vi "browseVariant.vi"(4 "Variant":variant caption="Value", 5 "Name":string, 6 "error in (no error)":errorcluster, 7 "ParentTag":string, 9 "VariantProbe.lvclass in":refnum<class "Failures_VariantTree__VP.lvclass">) -> (0 "error out":errorcluster, 3 "VariantProbe.lvclass out":refnum<class "Failures_VariantTree__VP.lvclass">)   [LabVIEW 2013, in "Failures_VariantTree__VP.lvclass"]
uses:
  Failures_VariantTree__VP.lvclass
  Failures_VariantTree__VP.lvclass/Failures_VariantTree__VP.ctl
  <vilib>/Utility/VariantDataType/VariantType.lvlib
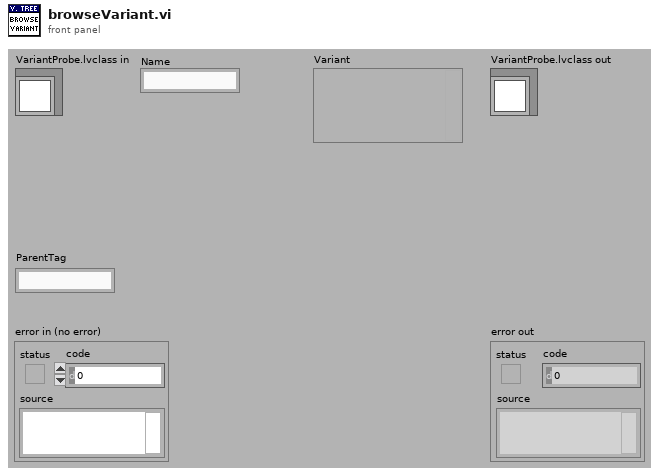
[diagram p1: front panel]
types:
  T1 = typedef "Type Descriptor Enumeration__ogtk.ctl" = enum8{"<Null>", "I8", "I16", "I32", "I64", "U8", "U16", "U32", "U64", "SGL", "DBL", "EXT", "CSG", "CDB", "CXT", "0x0F", "0x10", "0x11", "0x12", "0x13", "0x14", "Enum U8", "Enum U16", "Enum U32", "Enum U64", "SGL PQ", "DBL PQ", "EXT PQ", "CSG PQ", "CDB PQ", "CXT PQ", "0x1F", "0x20", "Boolean", "0x22", "0x23", "0x24", "0x25", "0x26", "0x27", "0x28", "0x29", "0x2A", "0x2B", "0x2C", "0x2D", "0x2E", "0x2F", "String", "0x31", "Path", "Pict", "0x34", "0x35", "0x36", "DAQ", "0x38", "0x39", "0x3A", "0x3B", "0x3C", "0x3D", "0x3E", "0x3F", "Array", "0x41", "0x42", "0x43", "0x44", "0x45", "0x46", "0x47", "0x48", "0x49", "0x4A", "0x4B", "0x4C", "0x4D", "0x4E", "0x4F", "Cluster", "0x51", "0x52", "Variant", "Waveform", "0x55", "0x56", "0x57", "0x58", "0x59", "0x5A", "0x5B", "0x5C", "0x5D", "0x5E", "0x5F", "0x60", "0x61", "0x62", "0x63", "0x64", "0x65", "0x66", "0x67", "0x68", "0x69", "0x6A", "0x6B", "0x6C", "0x6D", "0x6E", "0x6F", "Refnum"}
  T2 = typedef "Type Descriptor Header__ogtk.ctl" = cluster{"length":u16, "private":u8, "type":T1, "# elements":u16}
  T3 = typedef "Physical Units__ogtk.ctl" = cluster{"Base Units":enum16{"radian", "steradian", "second", "meter", "kilogram", "ampere", "kelvin", "mole", "candela"}, "Exponent":i16}
  T4 = enum16{"radian", "steradian", "second", "meter", "kilogram", "ampere", "kelvin", "mole", "candela"}
  T5 = typedef "VariantType.lvlib/RefnumType.ctl" = enum16{"NotARefnum", "UnknownRefnum", "Generic", "Datalog", "ByteStream", "Device", "Occurence", "TCPNetConnection", "Auto", "Menu", "Imaq", "Hardware", "DataSocket", "Visa", "IVI", "UDPNetConnection", "Notifier", "Queue", "Irda", "EventReg", "DotNet", "UserEvent", "Callback", "UNUSED_EMPTY_POSITION", "BlueToothNetConnection", "LVObjApp", "LVObjVI", "LVObjUnknown", "GenericClass", "UserDefinedRefnumTag", "DataValue", "RT FIFO", "TDMS File"}
  T6 = enum32{"invalid VI type", "Standard VI", "Control VI", "Global VI", "Polymorphic VI", "Configuration VI", "SubSystem", "Facade VI", "Method VI", "Statechart Diagram VI"}
  T7 = typedef "VariantType.lvlib/Type.ctl" = enum8{"Invalid Type", "Void", "I8", "I16", "I32", "I64", "U8", "U16", "U32", "U64", "Single Float", "Double Float", "Extended Float", "Single Complex", "Double Complex", "Extended Complex", "Enum U8", "Enum U16", "Enum U32", "Enum U64", "Single Float With Unit", "Double Float With Unit", "Extended Float With Unit", "Single Complex with Unit", "Double Complex with Unit", "Extended Complex with Unit", "Boolean", "String", "Path", "Picture", "Tag", "Array", "Cluster", "Variant", "LV Variant", "Waveform", "Timestamp", "Digital Waveform", "Digital Data", "ExpressData", "Refnum", "External Data", "VI", "Poly VI", "LabVIEW Class Instance", "Fixed Point"}
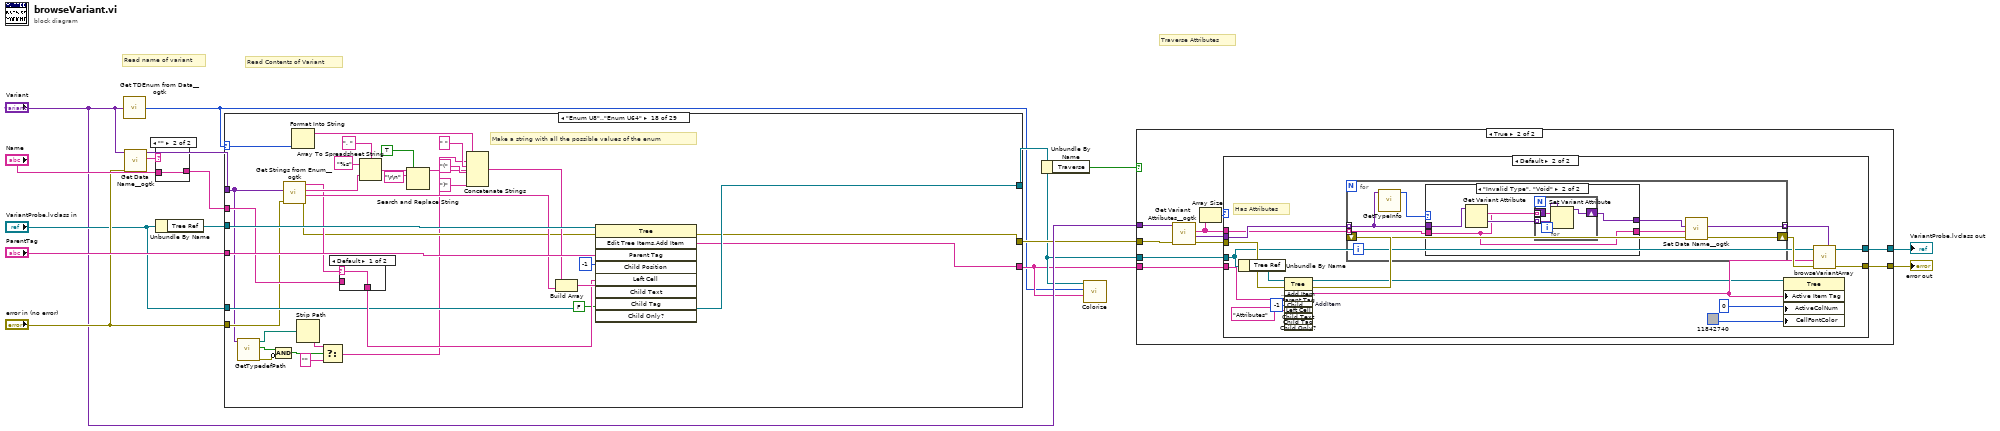
[diagram p0: block diagram]
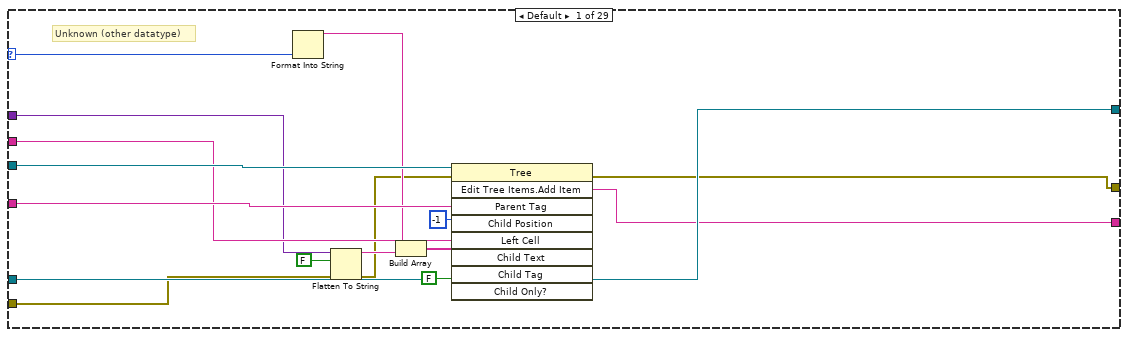
[diagram p6: hidden frame]
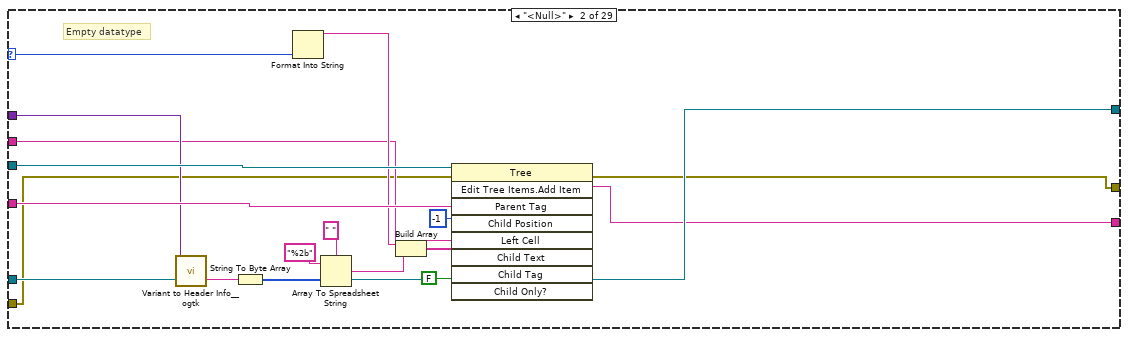
[diagram p7: hidden frame]
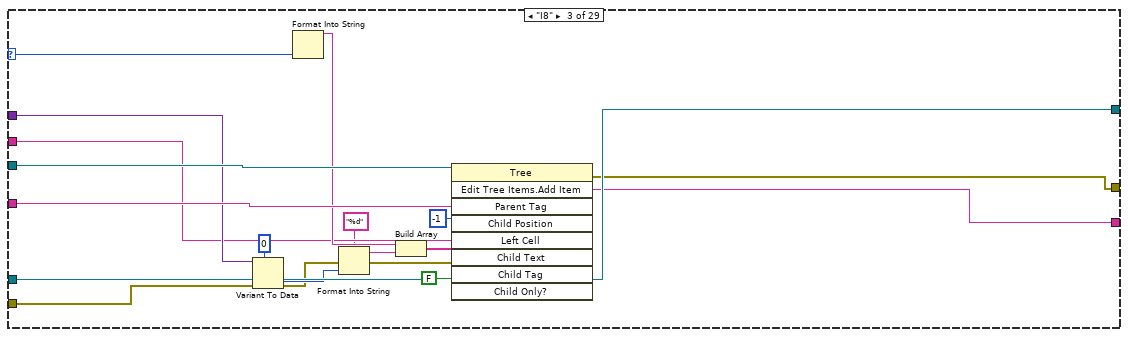
[diagram p8: hidden frame]
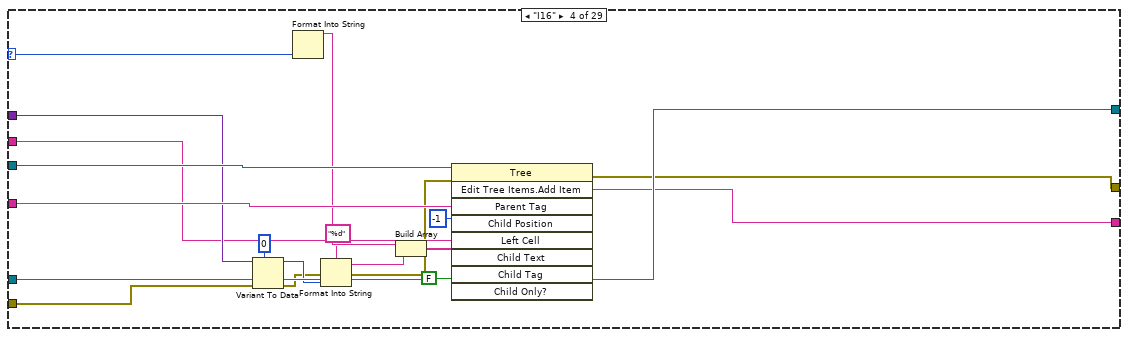
[diagram p9: hidden frame]
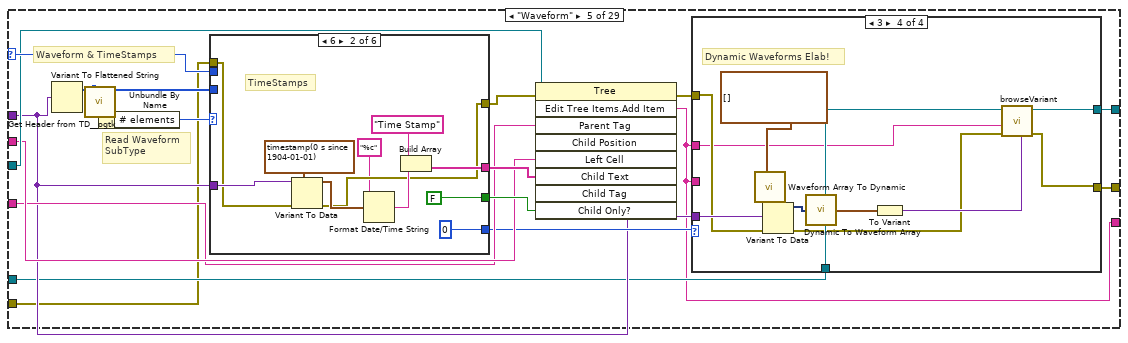
[diagram p10: hidden frame]
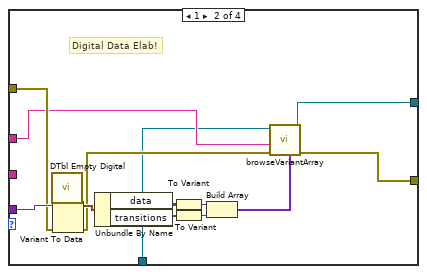
[diagram p12: hidden frame]
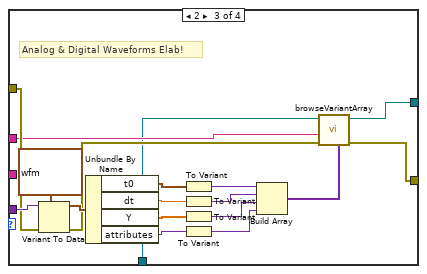
[diagram p13: hidden frame]
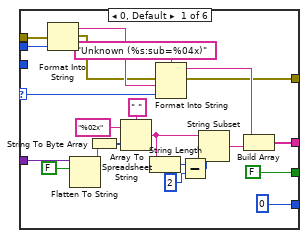
[diagram p14: hidden frame]
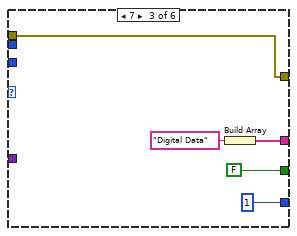
[diagram p15: hidden frame]
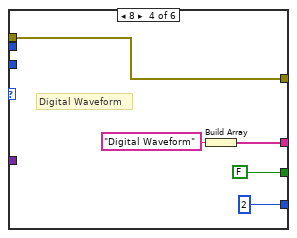
[diagram p16: hidden frame]
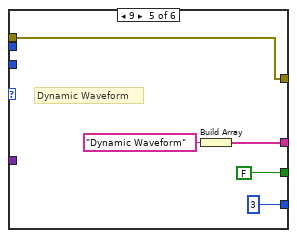
[diagram p17: hidden frame]
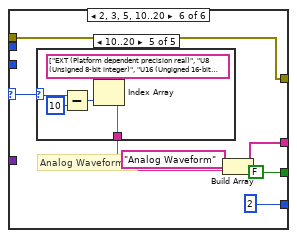
[diagram p18: hidden frame]
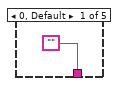
[diagram p19: hidden frame]
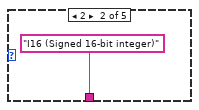
[diagram p20: hidden frame]
diagram:
  # "Traverse Attributes"
  # "Read Contents of Variant"
  # "Read name of variant"
  n1 = call <userlib>:"Get TDEnum from Data__ogtk.vi"("Data"="Variant") -> ("Type Descriptor Enumeration"=w1:T1)  [unwired: 4 in]
  n2 = call <userlib>:"Get Data Name__ogtk.vi"("error in (no error)"="error in (no error)", "Data"="Variant") -> ("Data Name"=w16:string, "Data dup"=w14:variant)  [unwired: 7 in, 1 out]
  n3 = case shown="\"\"" w16 {
    selector: w16 -> [w17 _]
    tunnel: [w17 w18] -> w13
    tunnel: "Name" -> [_ w18]
    frame Default {
    }
    frame "" {
    }
  }
  n4 = Unbundle By Name("VariantProbe.lvclass in") -> ("Tree Ref"=w4:refnum<vi>)
  n5 = case shown="\"Enum U8\"..\"Enum U64\"" w1 {
    selector: w1 -> [w34 w52 w71 w90 w105 w237 w256 w275 w294 w313 w332 w350 w368 w386 w404 w422 w440 w471 w504 w538 w572 w598 w614 w631 w647 _ _ _ w718]
    tunnel: w14 -> [w25 w41 w64 w83 w97 w230 w249 w268 w287 w306 w325 w339 w358 w376 w394 w412 w430 w448 w492 w526 w560 w587 w605 w622 w638 w659 w673 w703 w709]
    tunnel: w4 -> [w31 w49 w68 w87 w104 w234 w253 w272 w291 w310 w329 w347 w365 w383 w401 w419 w437 w475 w501 w535 w569 w595 w611 w628 w644 w669 w684 w708 w716]
    tunnel: "ParentTag" -> [w33 w51 w70 w89 w99 w236 w255 w274 w293 w312 w331 w349 w367 w385 w403 w421 w439 w474 w503 w537 w571 w597 w613 w630 w646 w668 w683 w707 w717]
    tunnel: w13 -> [w26 w40 w63 w82 w100 w229 w248 w267 w286 w305 w324 w340 w357 w375 w393 w411 w429 w457 w495 w529 w563 w586 w606 w621 w639 w660 w680 w702 w714]
    tunnel: "VariantProbe.lvclass in" -> [w23 w38 w61 w80 w96 w227 w246 w265 w284 w303 w322 w337 w355 w373 w391 w409 w427 w453 w485 w519 w553 w584 w603 w619 w636 w650 w678 w697 w713]
    tunnel: [w23 w38 w61 w80 w95 w227 w246 w265 w284 w303 w322 w337 w355 w373 w391 w409 w427 w453 w485 w519 w553 w584 w603 w619 w636 w649 w677 w695 w713] -> w3
    tunnel: "error in (no error)" -> [w22 w37 w59 w78 w94 w226 w244 w264 w283 w301 w321 w335 w354 w372 w390 w408 w425 w452 w484 w518 w552 w582 w601 w616 w635 w656 w675 w700 _]
    tunnel: [w20 w36 w60 w79 w92 w225 w245 w263 w282 w302 w314 w334 w352 w370 w388 w406 w424 w450 w479 w513 w547 w581 w600 w618 w633 w653 w676 w699 w712] -> w8
    tunnel: [w19 w35 w53 w72 w91 w219 w238 w257 w276 w295 w315 w333 w351 w369 w387 w405 w423 w449 w478 w512 w546 w580 w599 w615 w632 w648 w674 w694 w711] -> w2
    frame Default {
      # "Unknown (other datatype)"
      n6 = Format Into String(w34) -> (resulting string=w30:string)  [unwired: 3 in, 1 out]
      n7 = Flatten To String(anything=w25, prepend array or string size? (T)=FALSE, error in (no error)=w22) -> (data string=w28:string, error out=w21:errorcluster)  [unwired: 1 in, 1 out]
      n8 = Build Array(w30, w28) -> (w29:string[])
      n9 = invoke class="Tree" method="Edit Tree Items.Add Item"(reference=w31, error in=w21, "Parent Tag"=w33, "Child Position"=-1, "Left Cell"=w26, "Child Text"=w29, "Child Only?"=FALSE) -> (error out=w20:errorcluster, "Edit Tree Items:Add Item"=w19:string)  [unwired: 2 in, 7 out]
    }
    frame "<Null>" {
      # "Empty datatype"
      n10 = call <userlib>:"Variant to Header Info__ogtk.vi"("Variant"=w41) -> ("data string"=w43:string)  [unwired: 3 in, 2 out]
      n11 = String To Byte Array(string=w43) -> (unsigned byte array=w42:u8[])
      n12 = Format Into String(w52) -> (resulting string=w48:string)  [unwired: 3 in, 1 out]
      n13 = Array To Spreadsheet String(delimiter (Tab)=" ", array=w42, 3:"%2b" ("format string")) -> (spreadsheet string=w44:string)
      n14 = Build Array(w48, w44) -> (w47:string[])
      n15 = invoke class="Tree" method="Edit Tree Items.Add Item"(reference=w49, error in=w37, "Parent Tag"=w51, "Child Position"=-1, "Left Cell"=w40, "Child Text"=w47, "Child Only?"=FALSE) -> (error out=w36:errorcluster, "Edit Tree Items:Add Item"=w35:string)  [unwired: 2 in, 7 out]
    }
    frame "I8" {
      n16 = Variant To Data(error in=w59, type=i8 0, Variant=w64) -> (data=w58:i8, error out=w55:errorcluster)
      n17 = Format Into String(w71) -> (resulting string=w67:string)  [unwired: 3 in, 1 out]
      n18 = Format Into String(format string="%d", error in=w55, w58) -> (resulting string=w57:string, error out=w54:errorcluster)  [unwired: 1 in]
      n19 = Build Array(w67, w57) -> (w66:string[])
      n20 = invoke class="Tree" method="Edit Tree Items.Add Item"(reference=w68, error in=w54, "Parent Tag"=w70, "Child Position"=-1, "Left Cell"=w63, "Child Text"=w66, "Child Only?"=FALSE) -> (error out=w60:errorcluster, "Edit Tree Items:Add Item"=w53:string)  [unwired: 2 in, 7 out]
    }
    frame "I16" {
      n21 = Variant To Data(error in=w78, type=i16 0, Variant=w83) -> (data=w76:i16, error out=w75:errorcluster)
      n22 = Format Into String(w90) -> (resulting string=w86:string)  [unwired: 3 in, 1 out]
      n23 = Format Into String(format string="%d", error in=w75, w76) -> (resulting string=w73:string, error out=w74:errorcluster)  [unwired: 1 in]
      n24 = Build Array(w86, w73) -> (w85:string[])
      n25 = invoke class="Tree" method="Edit Tree Items.Add Item"(reference=w87, error in=w74, "Parent Tag"=w89, "Child Position"=-1, "Left Cell"=w82, "Child Text"=w85, "Child Only?"=FALSE) -> (error out=w79:errorcluster, "Edit Tree Items:Add Item"=w72:string)  [unwired: 2 in, 7 out]
    }
    frame "Waveform" {
      # "Read Waveform\nSubType"
      # "Waveform & TimeStamps"
      n26 = Variant To Flattened String(Variant=w97) -> (1:w108:i16[])  [unwired: 1 out]
      n27 = call <userlib>:"Get Header from TD__ogtk.vi"("Type Descriptor"=w108) -> ("Type Descriptor Header"=w106:T2)
      n28 = Unbundle By Name(w106) -> ("# elements"=w107:u16)
      n29 = case shown="6" w107 {
        selector: w107 -> [w163 _ _ _ _ w208]
        tunnel: [w165 w184 w191 w196 w201 w209] -> w102
        tunnel: w97 -> [w164 w186 _ _ _ _]
        tunnel: w108 -> [_ _ _ _ _ _]
        tunnel: [0 0 1 2 3 2] -> w98
        tunnel: [FALSE ("Child Only?") FALSE ("Child Only?") FALSE ("Child Only?") FALSE ("Child Only?") FALSE ("Child Only?") FALSE ("Child Only?")] -> w101
        tunnel: w105 -> [w159 _ _ _ _ _]
        tunnel: [w157 w178 w188 w193 w198 w203] -> w103
        tunnel: w94 -> [w155 w181 w188 w193 w198 w203]
        frame 0, Default {
          n30 = Format Into String(error in=w155, w159) -> (resulting string=w158:string, error out=w156:errorcluster)  [unwired: 2 in]
          n31 = Flatten To String(anything=w164, prepend array or string size? (T)=FALSE) -> (data string=w166:string)  [unwired: 2 in, 2 out]
          n32 = String To Byte Array(string=w166) -> (unsigned byte array=w160:u8[])
          n33 = Array To Spreadsheet String(delimiter (Tab)=" ", array=w160, 3:"%02x" ("format string")) -> (spreadsheet string=w172:string)
          n34 = String Length(string=w172) -> (length=w173:i32)
          n35 = Format Into String(format string="Unknown (%s:sub=%04x)", error in=w156, w158, w163) -> (resulting string=w169:string, error out=w157:errorcluster)  [unwired: 1 in]
          n36 = Subtract(x=w173, y=2) -> (x-y=w175:i32)
          n37 = String Subset(string=w172, length (rest)=w175) -> (substring=w176:string)  [unwired: 1 in]
          n38 = Build Array(w169, w176) -> (w165:string[])
        }
        frame 6 {
          # "TimeStamps"
          n39 = Variant To Data(error in=w181, type=timestamp(0 s since 1904-01-01), Variant=w186) -> (data=w179:timestamp, error out=w178:errorcluster)
          n40 = Format Date/Time String(time format string (%c)="%c" ("format string"), seconds (now)=w179) -> (date/time string=w180:string)  [unwired: 1 in]
          n41 = Build Array("Time Stamp" ("format string"), w180) -> (w184:string[])
        }
        frame 7 {
          n42 = Build Array("Digital Data" ("format string")) -> (w191:string[])
        }
        frame 8 {
          # "Digital Waveform"
          n43 = Build Array("Digital Waveform" ("format string")) -> (w196:string[])
        }
        frame 9 {
          # "Dynamic Waveform"
          n44 = Build Array("Dynamic Waveform" ("format string")) -> (w201:string[])
        }
        frame 2, 3, 5, 10..20 {
          # "Analog Waveform"
          n45 = case shown="10..20" w208 {
            selector: w208 -> [_ _ _ _ w216]
            tunnel: ["" "I16 (Signed 16-bit integer)" "DBL (Double 64-bit real)" "SGL (Single 32-bit real)" w218] -> w204
            frame 0, Default {
            }
            frame 2 {
            }
            frame 3 {
            }
            frame 5 {
            }
            frame 10..20 {
              n46 = Subtract(x=w216, y=u16 10) -> (x-y=w214:u16)
              n47 = Index Array(array=string[] ["EXT (Platform dependent precision real)", "U8 (Unsigned 8-bit integer)", "U16 (Ungigned 16-bit integer)", "U32 (Unsigned 32-bit integer)", "I8 (Signed 8-bit integer)", "I32 (Signed 32-bit integer)", "CSG (Single 32-bit complex real)", "CDB (Double 64-bit complex real)", "CXT (Extended complex real)", "I64 (Signed 64-bit integer)", "U64 (Unsigned 64-bit integer)"], index=w214) -> (element=w218:string)
            }
          }
          n48 = Build Array("Analog Waveform" ("format string"), w204) -> (w209:string[])
        }
      }
      n49 = invoke class="Tree" method="Edit Tree Items.Add Item"(reference=w104, error in=w103, "Parent Tag"=w99, "Left Cell"=w100, "Child Text"=w102, "Child Only?"=w101) -> (error out=w93:errorcluster, "Edit Tree Items:Add Item"=w91:string)  [unwired: 3 in, 7 out]
      n50 = case shown="3" w98 {
        tunnel: w91 -> [_ w114 w128 w147]
        tunnel: w97 -> [_ w124 w142 w150]
        tunnel: w91 -> [_ _ _ _]
        tunnel: w96 -> [w110 w112 w126 w148]
        tunnel: [w110 w111 w125 w145] -> w95
        tunnel: w93 -> [w109 w117 w131 w149]
        tunnel: [w109 w113 w127 w144] -> w92
        frame 0, Default {
          # "No further elaborations!"
        }
        frame 1 {
          # "Digital Data Elab!"
          n51 = call <vilib>:"DTbl Empty Digital.vi"() -> ("digital data"=w123:digitaldata)  [unwired: 5 in]
          n52 = Variant To Data(error in=w117, type=w123, Variant=w124) -> (data=w122:digitaldata, error out=w116:errorcluster)
          n53 = Unbundle By Name(w122) -> ("data"=w119:u8[][], "transitions"=w118:u32[])
          n54 = To Variant(anything=w119) -> (Variant=w121:variant)
          n55 = To Variant(anything=w118) -> (Variant=w120:variant)
          n56 = Build Array(w121, w120) -> (w115:variant[])
          n57 = call-dynamic "browseVariantArray.vi"("Array of Variants"=w115, "error in"=w116, "ParentTag"=w114, "VariantProbe.lvclass in"=w112) -> ("error out"=w113:errorcluster, "VariantProbe.lvclass out"=w111:refnum<class "Failures_VariantTree__VP.lvclass">)  [unwired: 4 in]
        }
        frame 2 {
          # "Analog & Digital Waveforms Elab!"
          n58 = Variant To Data(error in=w131, type=waveform(dbl) {"t0"=timestamp(0 s since 1904-01-01), "dt"=1.0, "Y"=[]} ("waveform"), Variant=w142) -> (data=w134:waveform(dbl), error out=w129:errorcluster)
          n59 = Unbundle By Name(w134) -> ("t0"=w136:timestamp, "dt"=w138:dbl, "Y"=w137:dbl[], "attributes"=w133:variant)
          n60 = To Variant(anything=w136) -> (Variant=w135:variant)
          n61 = To Variant(anything=w138) -> (Variant=w140:variant)
          n62 = To Variant(anything=w137) -> (Variant=w139:variant)
          n63 = To Variant(anything=w133) -> (Variant=w132:variant)
          n64 = Build Array(w135, w140, w139, w132) -> (w130:variant[])
          n65 = call-dynamic "browseVariantArray.vi"("Array of Variants"=w130, "error in"=w129, "ParentTag"=w128, "VariantProbe.lvclass in"=w126) -> ("error out"=w127:errorcluster, "VariantProbe.lvclass out"=w125:refnum<class "Failures_VariantTree__VP.lvclass">)  [unwired: 4 in]
        }
        frame 3 {
          # "Dynamic Waveforms Elab!"
          n66 = call <vilib>:"Waveform Array To Dynamic.vi"("Input"=waveform(dbl)[] []) -> ("Output"=w154:dynamicdata)  [unwired: 4 in]
          n67 = Variant To Data(error in=w149, type=w154, Variant=w150) -> (data=w153:dynamicdata, error out=w143:errorcluster)
          n68 = call <vilib>:"Dynamic To Waveform Array.vi"("Input"=w153) -> ("Output"=w151:waveform(dbl)[])  [unwired: 4 in]
          n69 = To Variant(anything=w151) -> (Variant=w146:variant)
          n70 = call-dynamic "browseVariant.vi"("Variant"=w146, "error in (no error)"=w143, "ParentTag"=w147, "VariantProbe.lvclass in"=w148) -> ("error out"=w144:errorcluster, "VariantProbe.lvclass out"=w145:refnum<class "Failures_VariantTree__VP.lvclass">)  [unwired: 4 in]
        }
      }
    }
    frame "I32" {
      n71 = Variant To Data(error in=w226, type=0, Variant=w230) -> (data=w222:i32, error out=w223:errorcluster)
      n72 = Format Into String(w237) -> (resulting string=w233:string)  [unwired: 3 in, 1 out]
      n73 = Format Into String(format string="%d", error in=w223, w222) -> (resulting string=w220:string, error out=w221:errorcluster)  [unwired: 1 in]
      n74 = Build Array(w233, w220) -> (w232:string[])
      n75 = invoke class="Tree" method="Edit Tree Items.Add Item"(reference=w234, error in=w221, "Parent Tag"=w236, "Child Position"=-1, "Left Cell"=w229, "Child Text"=w232, "Child Only?"=FALSE) -> (error out=w225:errorcluster, "Edit Tree Items:Add Item"=w219:string)  [unwired: 2 in, 7 out]
    }
    frame "I64" {
      # "I64"
      n76 = Variant To Data(error in=w244, type=i64 0, Variant=w249) -> (data=w241:i64, error out=w242:errorcluster)
      n77 = Format Into String(w256) -> (resulting string=w252:string)  [unwired: 3 in, 1 out]
      n78 = Format Into String(format string="%d", error in=w242, w241) -> (resulting string=w240:string, error out=w239:errorcluster)  [unwired: 1 in]
      n79 = Build Array(w252, w240) -> (w251:string[])
      n80 = invoke class="Tree" method="Edit Tree Items.Add Item"(reference=w253, error in=w239, "Parent Tag"=w255, "Child Position"=-1, "Left Cell"=w248, "Child Text"=w251, "Child Only?"=FALSE) -> (error out=w245:errorcluster, "Edit Tree Items:Add Item"=w238:string)  [unwired: 2 in, 7 out]
    }
    frame "U8" {
      n81 = Variant To Data(error in=w264, type=u8 0, Variant=w268) -> (data=w261:u8, error out=w260:errorcluster)
      n82 = Format Into String(w275) -> (resulting string=w271:string)  [unwired: 3 in, 1 out]
      n83 = Format Into String(format string="%d", error in=w260, w261) -> (resulting string=w258:string, error out=w259:errorcluster)  [unwired: 1 in]
      n84 = Build Array(w271, w258) -> (w270:string[])
      n85 = invoke class="Tree" method="Edit Tree Items.Add Item"(reference=w272, error in=w259, "Parent Tag"=w274, "Child Position"=-1, "Left Cell"=w267, "Child Text"=w270, "Child Only?"=FALSE) -> (error out=w263:errorcluster, "Edit Tree Items:Add Item"=w257:string)  [unwired: 2 in, 7 out]
    }
    frame "U16" {
      n86 = Variant To Data(error in=w283, type=u16 0, Variant=w287) -> (data=w277:u16, error out=w278:errorcluster)
      n87 = Format Into String(w294) -> (resulting string=w290:string)  [unwired: 3 in, 1 out]
      n88 = Format Into String(format string="%d", error in=w278, w277) -> (resulting string=w280:string, error out=w279:errorcluster)  [unwired: 1 in]
      n89 = Build Array(w290, w280) -> (w289:string[])
      n90 = invoke class="Tree" method="Edit Tree Items.Add Item"(reference=w291, error in=w279, "Parent Tag"=w293, "Child Position"=-1, "Left Cell"=w286, "Child Text"=w289, "Child Only?"=FALSE) -> (error out=w282:errorcluster, "Edit Tree Items:Add Item"=w276:string)  [unwired: 2 in, 7 out]
    }
    frame "U32" {
      n91 = Variant To Data(error in=w301, type=u32 0, Variant=w306) -> (data=w299:u32, error out=w298:errorcluster)
      n92 = Format Into String(w313) -> (resulting string=w309:string)  [unwired: 3 in, 1 out]
      n93 = Format Into String(format string="%d", error in=w298, w299) -> (resulting string=w296:string, error out=w297:errorcluster)  [unwired: 1 in]
      n94 = Build Array(w309, w296) -> (w308:string[])
      n95 = invoke class="Tree" method="Edit Tree Items.Add Item"(reference=w310, error in=w297, "Parent Tag"=w312, "Child Position"=-1, "Left Cell"=w305, "Child Text"=w308, "Child Only?"=FALSE) -> (error out=w302:errorcluster, "Edit Tree Items:Add Item"=w295:string)  [unwired: 2 in, 7 out]
    }
    frame "U64" {
      # "U64"
      n96 = Variant To Data(error in=w321, type=u64 0, Variant=w325) -> (data=w319:u64, error out=w318:errorcluster)
      n97 = Format Into String(w332) -> (resulting string=w328:string)  [unwired: 3 in, 1 out]
      n98 = Format Into String(format string="%d", error in=w318, w319) -> (resulting string=w316:string, error out=w317:errorcluster)  [unwired: 1 in]
      n99 = Build Array(w328, w316) -> (w327:string[])
      n100 = invoke class="Tree" method="Edit Tree Items.Add Item"(reference=w329, error in=w317, "Parent Tag"=w331, "Child Position"=-1, "Left Cell"=w324, "Child Text"=w327, "Child Only?"=FALSE) -> (error out=w314:errorcluster, "Edit Tree Items:Add Item"=w315:string)  [unwired: 2 in, 7 out]
    }
    frame "SGL" {
      n101 = Variant To Data(error in=w335, type=sgl 0.0, Variant=w339) -> (data=w342:sgl, error out=w336:errorcluster)
      n102 = Format Into String(w350) -> (resulting string=w346:string)  [unwired: 3 in, 1 out]
      n103 = Format Value(format string="%f", value (0)=w342) -> (output string=w341:string)  [unwired: 1 in]
      n104 = Build Array(w346, w341) -> (w345:string[])
      n105 = invoke class="Tree" method="Edit Tree Items.Add Item"(reference=w347, error in=w336, "Parent Tag"=w349, "Child Position"=-1, "Left Cell"=w340, "Child Text"=w345, "Child Only?"=FALSE) -> (error out=w334:errorcluster, "Edit Tree Items:Add Item"=w333:string)  [unwired: 2 in, 7 out]
    }
    frame "DBL" {
      n106 = Variant To Data(error in=w354, type=0.0, Variant=w358) -> (data=w360:dbl, error out=w353:errorcluster)
      n107 = Format Into String(w368) -> (resulting string=w364:string)  [unwired: 3 in, 1 out]
      n108 = Format Value(format string="%f", value (0)=w360) -> (output string=w359:string)  [unwired: 1 in]
      n109 = Build Array(w364, w359) -> (w363:string[])
      n110 = invoke class="Tree" method="Edit Tree Items.Add Item"(reference=w365, error in=w353, "Parent Tag"=w367, "Child Position"=-1, "Left Cell"=w357, "Child Text"=w363, "Child Only?"=FALSE) -> (error out=w352:errorcluster, "Edit Tree Items:Add Item"=w351:string)  [unwired: 2 in, 7 out]
    }
    frame "EXT" {
      n111 = Variant To Data(error in=w372, type=ext 0.0, Variant=w376) -> (data=w378:ext, error out=w371:errorcluster)
      n112 = Format Into String(w386) -> (resulting string=w382:string)  [unwired: 3 in, 1 out]
      n113 = Format Value(format string="%f", value (0)=w378) -> (output string=w377:string)  [unwired: 1 in]
      n114 = Build Array(w382, w377) -> (w381:string[])
      n115 = invoke class="Tree" method="Edit Tree Items.Add Item"(reference=w383, error in=w371, "Parent Tag"=w385, "Child Position"=-1, "Left Cell"=w375, "Child Text"=w381, "Child Only?"=FALSE) -> (error out=w370:errorcluster, "Edit Tree Items:Add Item"=w369:string)  [unwired: 2 in, 7 out]
    }
    frame "CSG" {
      n116 = Variant To Data(error in=w390, type=csg 0.0+0.0i, Variant=w394) -> (data=w396:csg, error out=w389:errorcluster)
      n117 = Format Into String(w404) -> (resulting string=w400:string)  [unwired: 3 in, 1 out]
      n118 = Format Value(format string="%f", value (0)=w396) -> (output string=w395:string)  [unwired: 1 in]
      n119 = Build Array(w400, w395) -> (w399:string[])
      n120 = invoke class="Tree" method="Edit Tree Items.Add Item"(reference=w401, error in=w389, "Parent Tag"=w403, "Child Position"=-1, "Left Cell"=w393, "Child Text"=w399, "Child Only?"=FALSE) -> (error out=w388:errorcluster, "Edit Tree Items:Add Item"=w387:string)  [unwired: 2 in, 7 out]
    }
    frame "CDB" {
      n121 = Variant To Data(error in=w408, type=cdb 0.0+0.0i, Variant=w412) -> (data=w414:cdb, error out=w407:errorcluster)
      n122 = Format Into String(w422) -> (resulting string=w418:string)  [unwired: 3 in, 1 out]
      n123 = Format Value(format string="%f", value (0)=w414) -> (output string=w413:string)  [unwired: 1 in]
      n124 = Build Array(w418, w413) -> (w417:string[])
      n125 = invoke class="Tree" method="Edit Tree Items.Add Item"(reference=w419, error in=w407, "Parent Tag"=w421, "Child Position"=-1, "Left Cell"=w411, "Child Text"=w417, "Child Only?"=FALSE) -> (error out=w406:errorcluster, "Edit Tree Items:Add Item"=w405:string)  [unwired: 2 in, 7 out]
    }
    frame "CXT" {
      n126 = Variant To Data(error in=w425, type=cxt 0.0+0.0i, Variant=w430) -> (data=w432:cxt, error out=w426:errorcluster)
      n127 = Format Into String(w440) -> (resulting string=w436:string)  [unwired: 3 in, 1 out]
      n128 = Format Value(format string="%f", value (0)=w432) -> (output string=w431:string)  [unwired: 1 in]
      n129 = Build Array(w436, w431) -> (w435:string[])
      n130 = invoke class="Tree" method="Edit Tree Items.Add Item"(reference=w437, error in=w426, "Parent Tag"=w439, "Child Position"=-1, "Left Cell"=w429, "Child Text"=w435, "Child Only?"=FALSE) -> (error out=w424:errorcluster, "Edit Tree Items:Add Item"=w423:string)  [unwired: 2 in, 7 out]
    }
    frame "Enum U8".."Enum U64" {
      # "Make a string with all the possible values of the enum"
      n131 = call <vilib>:"GetTypedefPath.vi"("Variant"=w448) -> ("error out"=w446:errorcluster, "HasPath"=w447:bool, "TypedefPath"=w444:path)  [unwired: 8 in]
      n132 = Compound Arithmetic op=AND(w447, invert w446) -> (w445:bool)
      n133 = call <userlib>:"Get Strings from Enum__ogtk.vi"("error in (no error)"=w452, "Enum"=w448) -> ("error out"=w451:errorcluster, "String Value"=w470:string, "Enum Strings"=w469:string[], "Enum Name"=w458:string)  [unwired: 6 in]
      n134 = Format Into String(w471) -> (resulting string=w467:string)  [unwired: 3 in, 1 out]
      n135 = Strip Path(path=w444) -> (name=w443:string)  [unwired: 1 out]
      n136 = Select(t=w443, s=w445, f="") -> (s? t:f=w441:string)
      n137 = case shown="Default" w458 {
        selector: w458 -> [w476 _]
        tunnel: [w476 w477] -> w456
        tunnel: w457 -> [_ w477]
        frame Default {
        }
        frame "" {
        }
      }
      n138 = Array To Spreadsheet String(delimiter (Tab)=", ", array=w469, 3:"%s" ("format string")) -> (spreadsheet string=w460:string)
      n139 = Search and Replace String(replace all?=TRUE ("replace all? (F)"), input string=w460, search string="\r\n") -> (result string=w459:string)  [unwired: 5 in, 3 out]
      n140 = Concatenate Strings(w467, w441, " " ("string"), "(" ("string"), w459, ")" ("string")) -> (w454:string)
      n141 = Build Array(w454, w470) -> (w472:string[])
      n142 = invoke class="Tree" method="Edit Tree Items.Add Item"(reference=w475, error in=w451, "Parent Tag"=w474, "Child Position"=-1, "Left Cell"=w456, "Child Text"=w472, "Child Only?"=FALSE) -> (error out=w450:errorcluster, "Edit Tree Items:Add Item"=w449:string)  [unwired: 2 in, 7 out]
    }
    frame "SGL PQ" {
      # "strip last '*'"
      # "Add physical quantity to string"
      n143 = call <userlib>:"Get Physical Units__ogtk.vi"("error in (no error)"=w484, "Float or Array of Floats"=w492) -> ("error out"=w483:errorcluster, "Physical Units"=w491:T3[])  [unwired: 8 in]
      n144 = call <userlib>:"Strip Units__ogtk.vi"("error in (no error)"=w483, "Number or 1D array with units"=w492) -> ("error out"=w482:errorcluster, "Pure Number(s) (base units)"=w493:variant)  [unwired: 8 in]
      n145 = for {
        tunnel: w491 -> [w511] mode=indexing
        tunnel: [w507] -> w490 mode=indexing
        shift-right: [w505] -> w481
        shift-left: w482 -> [w506]
        n146 = Unbundle(w511) -> ("Base Units"=w510:T4, "Exponent"=w509:i16)
        n147 = Format Into String(format string="%s ^(%d)*", error in=w506, w510, w509) -> (resulting string=w507:string, error out=w505:errorcluster)  [unwired: 1 in]
      }
      n148 = Format Into String(w504) -> (resulting string=w500:string)  [unwired: 3 in, 1 out]
      n149 = Variant To Data(error in=w481, type=sgl 0.0, Variant=w493) -> (data=w496:sgl, error out=w480:errorcluster)
      n150 = Format Value(format string="%f", value (0)=w496) -> (output string=w487:string)  [unwired: 1 in]
      n151 = Concatenate Strings(w487, w490) -> (w489:string)
      n152 = call <userlib>:"Slice String__ogtk.vi"("slice"=":-1", "string"=w489) -> ("substring"=w486:string)  [unwired: 5 in]
      n153 = Build Array(w500, w486) -> (w499:string[])
      n154 = invoke class="Tree" method="Edit Tree Items.Add Item"(reference=w501, error in=w480, "Parent Tag"=w503, "Child Position"=-1, "Left Cell"=w495, "Child Text"=w499, "Child Only?"=FALSE) -> (error out=w479:errorcluster, "Edit Tree Items:Add Item"=w478:string)  [unwired: 2 in, 7 out]
    }
    frame "DBL PQ" {
      # "strip last '*'"
      # "Add physical quantity to string"
      n155 = call <userlib>:"Get Physical Units__ogtk.vi"("error in (no error)"=w518, "Float or Array of Floats"=w526) -> ("error out"=w517:errorcluster, "Physical Units"=w525:T3[])  [unwired: 8 in]
      n156 = call <userlib>:"Strip Units__ogtk.vi"("error in (no error)"=w517, "Number or 1D array with units"=w526) -> ("error out"=w516:errorcluster, "Pure Number(s) (base units)"=w527:variant)  [unwired: 8 in]
      n157 = for {
        tunnel: w525 -> [w545] mode=indexing
        tunnel: [w541] -> w524 mode=indexing
        shift-right: [w539] -> w515
        shift-left: w516 -> [w540]
        n158 = Unbundle(w545) -> ("Base Units"=w544:T4, "Exponent"=w543:i16)
        n159 = Format Into String(format string="%s ^(%d)*", error in=w540, w544, w543) -> (resulting string=w541:string, error out=w539:errorcluster)  [unwired: 1 in]
      }
      n160 = Format Into String(w538) -> (resulting string=w534:string)  [unwired: 3 in, 1 out]
      n161 = Variant To Data(error in=w515, type=0.0, Variant=w527) -> (data=w530:dbl, error out=w514:errorcluster)
      n162 = Format Value(format string="%f", value (0)=w530) -> (output string=w521:string)  [unwired: 1 in]
      n163 = Concatenate Strings(w521, w524) -> (w523:string)
      n164 = call <userlib>:"Slice String__ogtk.vi"("slice"=":-1", "string"=w523) -> ("substring"=w520:string)  [unwired: 5 in]
      n165 = Build Array(w534, w520) -> (w533:string[])
      n166 = invoke class="Tree" method="Edit Tree Items.Add Item"(reference=w535, error in=w514, "Parent Tag"=w537, "Child Position"=-1, "Left Cell"=w529, "Child Text"=w533, "Child Only?"=FALSE) -> (error out=w513:errorcluster, "Edit Tree Items:Add Item"=w512:string)  [unwired: 2 in, 7 out]
    }
    frame "EXT PQ" {
      # "strip last '*'"
      # "Add physical quantity to string"
      n167 = call <userlib>:"Get Physical Units__ogtk.vi"("error in (no error)"=w552, "Float or Array of Floats"=w560) -> ("error out"=w551:errorcluster, "Physical Units"=w559:T3[])  [unwired: 8 in]
      n168 = call <userlib>:"Strip Units__ogtk.vi"("error in (no error)"=w551, "Number or 1D array with units"=w560) -> ("error out"=w550:errorcluster, "Pure Number(s) (base units)"=w561:variant)  [unwired: 8 in]
      n169 = for {
        tunnel: w559 -> [w579] mode=indexing
        tunnel: [w575] -> w558 mode=indexing
        shift-right: [w573] -> w549
        shift-left: w550 -> [w574]
        n170 = Unbundle(w579) -> ("Base Units"=w578:T4, "Exponent"=w577:i16)
        n171 = Format Into String(format string="%s ^(%d)*", error in=w574, w578, w577) -> (resulting string=w575:string, error out=w573:errorcluster)  [unwired: 1 in]
      }
      n172 = Format Into String(w572) -> (resulting string=w568:string)  [unwired: 3 in, 1 out]
      n173 = Variant To Data(error in=w549, type=ext 0.0, Variant=w561) -> (data=w564:ext, error out=w548:errorcluster)
      n174 = Format Value(format string="%f", value (0)=w564) -> (output string=w555:string)  [unwired: 1 in]
      n175 = Concatenate Strings(w555, w558) -> (w557:string)
      n176 = call <userlib>:"Slice String__ogtk.vi"("slice"=":-1", "string"=w557) -> ("substring"=w554:string)  [unwired: 5 in]
      n177 = Build Array(w568, w554) -> (w567:string[])
      n178 = invoke class="Tree" method="Edit Tree Items.Add Item"(reference=w569, error in=w548, "Parent Tag"=w571, "Child Position"=-1, "Left Cell"=w563, "Child Text"=w567, "Child Only?"=FALSE) -> (error out=w547:errorcluster, "Edit Tree Items:Add Item"=w546:string)  [unwired: 2 in, 7 out]
    }
    frame "Boolean" {
      n179 = Variant To Data(error in=w582, type=TRUE, Variant=w587) -> (data=w591:bool, error out=w583:errorcluster)
      n180 = Format Into String(w598) -> (resulting string=w594:string)  [unwired: 3 in, 1 out]
      n181 = Append True/False String(1:w591, 2:"False" ("false string"), 3:"True" ("true string")) -> (0:w590:string)  [unwired: 1 in]
      n182 = Build Array(w594, w590) -> (w593:string[])
      n183 = invoke class="Tree" method="Edit Tree Items.Add Item"(reference=w595, error in=w583, "Parent Tag"=w597, "Child Position"=-1, "Left Cell"=w586, "Child Text"=w593, "Child Only?"=FALSE) -> (error out=w581:errorcluster, "Edit Tree Items:Add Item"=w580:string)  [unwired: 2 in, 7 out]
    }
    frame "String", "DAQ" {
      n184 = Variant To Data(error in=w601, type="", Variant=w605) -> (data=w607:string, error out=w602:errorcluster)
      n185 = Format Into String(w614) -> (resulting string=w610:string)  [unwired: 3 in, 1 out]
      n186 = Build Array(w610, w607) -> (w609:string[])
      n187 = invoke class="Tree" method="Edit Tree Items.Add Item"(reference=w611, error in=w602, "Parent Tag"=w613, "Child Position"=-1, "Left Cell"=w606, "Child Text"=w609, "Child Only?"=FALSE) -> (error out=w600:errorcluster, "Edit Tree Items:Add Item"=w599:string)  [unwired: 2 in, 7 out]
    }
    frame "Path" {
      n188 = Variant To Data(error in=w616, type=path "", Variant=w622) -> (data=w624:path, error out=w617:errorcluster)
      n189 = Format Into String(w631) -> (resulting string=w627:string)  [unwired: 3 in, 1 out]
      n190 = Path To String(path=w624) -> (string=w623:string)
      n191 = Build Array(w627, w623) -> (w626:string[])
      n192 = invoke class="Tree" method="Edit Tree Items.Add Item"(reference=w628, error in=w617, "Parent Tag"=w630, "Child Position"=-1, "Left Cell"=w621, "Child Text"=w626, "Child Only?"=FALSE) -> (error out=w618:errorcluster, "Edit Tree Items:Add Item"=w615:string)  [unwired: 2 in, 7 out]
    }
    frame "Pict" {
      # "Add pict information in binary form"
      # "Unknown (other datatype)"
      n193 = Format Into String(w647) -> (resulting string=w643:string)  [unwired: 3 in, 1 out]
      n194 = Flatten To String(anything=w638, prepend array or string size? (T)=FALSE, error in (no error)=w635) -> (data string=w641:string, error out=w634:errorcluster)  [unwired: 1 in, 1 out]
      n195 = Build Array(w643, w641) -> (w642:string[])
      n196 = invoke class="Tree" method="Edit Tree Items.Add Item"(reference=w644, error in=w634, "Parent Tag"=w646, "Child Position"=-1, "Left Cell"=w639, "Child Text"=w642, "Child Only?"=FALSE) -> (error out=w633:errorcluster, "Edit Tree Items:Add Item"=w632:string)  [unwired: 2 in, 7 out]
    }
    frame "Array" {
      # "Load Same VI recursive, just one time"
      # "New branch for array"
      n197 = call <userlib>:"Reshape Array to 1D VArray__ogtk.vi"("error in (no error)"=w656, "MultiD Array"=w659) -> ("error out"=w655:errorcluster, "Size(s)"=w658:u32[], "1D VArray"=w657:variant)  [unwired: 7 in]
      n198 = Multiply Array Elements(1:w658) -> (0:w661:u32)
      n199 = Format Into String(format string="[%d]", initial string="Array", w661) -> (resulting string=w663:string)  [unwired: 1 in, 1 out]
      n200 = Build Array(w663) -> (w662:string[])
      n201 = invoke class="Tree" method="Edit Tree Items.Add Item"(reference=w669, error in=w655, "Parent Tag"=w668, "Child Position"=-1, "Left Cell"=w660, "Child Text"=w662, "Child Only?"=FALSE) -> (error out=w654:errorcluster, "Edit Tree Items:Add Item"=w648:string)  [unwired: 2 in, 7 out]
      n202 = call <userlib>:"Array to Array of VData__ogtk.vi"("error in (no error)"=w654, "MultiD Array"=w657) -> ("error out"=w652:errorcluster, "1D Array of Variants"=w651:variant[])  [unwired: 8 in]
      n203 = call-dynamic "browseVariantArray.vi"("Array of Variants"=w651, "error in"=w652, "ParentTag"=w648, "VariantProbe.lvclass in"=w650) -> ("error out"=w653:errorcluster, "VariantProbe.lvclass out"=w649:refnum<class "Failures_VariantTree__VP.lvclass">)  [unwired: 4 in]
    }
    frame "Cluster" {
      # "Load Same VI recursive"
      # "New branch for cluster"
      n204 = invoke class="Tree" method="Edit Tree Items.Add Item"(reference=w684, error in=w675, "Parent Tag"=w683, "Child Position"=-1, "Left Cell"=w680, "Child Text"=string[] ["Cluster"], "Child Only?"=FALSE) -> (error out=w672:errorcluster, "Edit Tree Items:Add Item"=w674:string)  [unwired: 2 in, 7 out]
      n205 = call <userlib>:"Cluster to Array of VData__ogtk.vi"("error in (no error)"=w672, "Cluster"=w673) -> ("error out"=w671:errorcluster, "Array of VData"=w670:variant[])  [unwired: 8 in]
      n206 = for {
        tunnel: w674 -> [w693]
        shift-right: [w691] -> w677
        shift-left: w678 -> [w692]
        shift-right: [w690] -> w676
        shift-left: w671 -> [w685]
        tunnel: w670 -> [w688] mode=indexing
        n207 = call <userlib>:"Get Data Name__ogtk.vi"("error in (no error)"=w685, "Data"=w688) -> ("error out"=w686:errorcluster, "Data Name"=w689:string, "Data dup"=w687:variant)  [unwired: 7 in]
        n208 = call-dynamic "browseVariant.vi"("Variant"=w687, "Name"=w689, "error in (no error)"=w686, "ParentTag"=w693, "VariantProbe.lvclass in"=w692) -> ("error out"=w690:errorcluster, "VariantProbe.lvclass out"=w691:refnum<class "Failures_VariantTree__VP.lvclass">)  [unwired: 3 in]
      }
    }
    frame "Variant" {
      # "New Branch for variant"
      # "Load Same VI recursive"
      n209 = call <userlib>:"Unwrap VVariant__ogtk.vi"("error in (no error)"=w700, "VVariant"=w703) -> ("error out"=w701:errorcluster, "Variant"=w696:variant)  [unwired: 8 in]
      n210 = invoke class="Tree" method="Edit Tree Items.Add Item"(reference=w708, error in=w701, "Parent Tag"=w707, "Child Position"=-1, "Left Cell"=w702, "Child Text"=string[] ["Variant"], "Child Only?"=FALSE) -> (error out=w698:errorcluster, "Edit Tree Items:Add Item"=w694:string)  [unwired: 2 in, 7 out]
      n211 = call-dynamic "browseVariant.vi"("Variant"=w696, "error in (no error)"=w698, "ParentTag"=w694, "VariantProbe.lvclass in"=w697) -> ("error out"=w699:errorcluster, "VariantProbe.lvclass out"=w695:refnum<class "Failures_VariantTree__VP.lvclass">)  [unwired: 4 in]
    }
    frame "Refnum" {
      n212 = call <vilib>:"GetRefnumInfo.vi"("Variant"=w709) -> ("ReferenceType"=w710:T5)  [unwired: 7 in, 3 out]
      n213 = Format Into String(w718) -> (resulting string=w715:string)  [unwired: 3 in, 1 out]
      n214 = case shown="\"GenericClass\"" w710 {
        tunnel: w717 -> [w734 w746 w763 w779 w793]
        tunnel: w716 -> [w732 w744 w761 w777 w791]
        tunnel: w715 -> [w731 w743 w760 w776 w790]
        tunnel: w714 -> [w729 w741 w758 w774 w788]
        tunnel: [w725 w737 w754 w770 w784] -> w712
        tunnel: [w724 w736 w753 w769 w783] -> w711
        tunnel: w710 -> [w723 w735 w752 w768 w782]
        tunnel: w709 -> [w722 _ w751 w767 w781]
        frame "Generic" {
          w721 = refnum<vi> refnum  # Generic
          n215 = Variant To Data(type=w721, Variant=w722) -> (data=w720:refnum<vi>)  [unwired: 1 in, 1 out]
          n216 = property class="Gen"(reference=w720) -> ("ClassName"=w719:string)  [unwired: 1 in, 2 out]
          n217 = Format Into String(format string="%s (%s)", w723, w719) -> (resulting string=w726:string)  [unwired: 2 in, 1 out]
          n218 = Build Array(w731, w726) -> (w730:string[])
          n219 = invoke class="Tree" method="Edit Tree Items.Add Item"(reference=w732, "Parent Tag"=w734, "Child Position"=-1, "Left Cell"=w729, "Child Text"=w730, "Child Only?"=FALSE) -> (error out=w725:errorcluster, "Edit Tree Items:Add Item"=w724:string)  [unwired: 3 in, 7 out]
        }
        frame Default {
          n220 = Format Into String(format string="%s", w735) -> (resulting string=w738:string)  [unwired: 2 in, 1 out]
          n221 = Build Array(w743, w738) -> (w742:string[])
          n222 = invoke class="Tree" method="Edit Tree Items.Add Item"(reference=w744, "Parent Tag"=w746, "Child Position"=-1, "Left Cell"=w741, "Child Text"=w742, "Child Only?"=FALSE) -> (error out=w737:errorcluster, "Edit Tree Items:Add Item"=w736:string)  [unwired: 3 in, 7 out]
        }
        frame "LVObjVI" {
          n223 = Variant To Data(type=refnum<vi> refnum ("vi reference"), Variant=w751) -> (data=w750:refnum<vi>)  [unwired: 1 in, 1 out]
          n224 = property class="VI"(reference=w750) -> ("VIType"=w749:T6, "Name"=w748:string)  [unwired: 1 in, 2 out]
          n225 = Format Into String(format string="%s (%s, %s)", w752, w749, w748) -> (resulting string=w755:string)  [unwired: 2 in, 1 out]
          n226 = Build Array(w760, w755) -> (w759:string[])
          n227 = invoke class="Tree" method="Edit Tree Items.Add Item"(reference=w761, "Parent Tag"=w763, "Child Position"=-1, "Left Cell"=w758, "Child Text"=w759, "Child Only?"=FALSE) -> (error out=w754:errorcluster, "Edit Tree Items:Add Item"=w753:string)  [unwired: 3 in, 7 out]
        }
        frame "LVObjApp" {
          n228 = control-ref of="This Application"() -> (w764:refnum<vi>)
          n229 = Variant To Data(type=w764, Variant=w767) -> (data=w766:refnum<vi>)  [unwired: 1 in, 1 out]
          n230 = property class="App"(reference=w766) -> ("App.Name"=w765:string)  [unwired: 1 in, 2 out]
          n231 = Format Into String(format string="%s (%s)", w768, w765) -> (resulting string=w771:string)  [unwired: 2 in, 1 out]
          n232 = Build Array(w776, w771) -> (w775:string[])
          n233 = invoke class="Tree" method="Edit Tree Items.Add Item"(reference=w777, "Parent Tag"=w779, "Child Position"=-1, "Left Cell"=w774, "Child Text"=w775, "Child Only?"=FALSE) -> (error out=w770:errorcluster, "Edit Tree Items:Add Item"=w769:string)  [unwired: 3 in, 7 out]
        }
        frame "GenericClass" {
          n234 = call <vilib>:"GetLVClassInfo.vi"("Variant"=w781) -> ("LV Class File Name"=w780:string)  [unwired: 8 in, 2 out]
          n235 = Format Into String(format string="%s (%s)", w782, w780) -> (resulting string=w785:string)  [unwired: 2 in, 1 out]
          n236 = Build Array(w790, w785) -> (w789:string[])
          n237 = invoke class="Tree" method="Edit Tree Items.Add Item"(reference=w791, "Parent Tag"=w793, "Child Position"=-1, "Left Cell"=w788, "Child Text"=w789, "Child Only?"=FALSE) -> (error out=w784:errorcluster, "Edit Tree Items:Add Item"=w783:string)  [unwired: 3 in, 7 out]
        }
      }
    }
  }
  n238 = Unbundle By Name(w3) -> ("Traverse"=w5:bool)
  n239 = call "Colorize.vi"("Tag"=w2, "Type Descriptor Enum"=w1, "VariantTree in"=w3) -> ()  [unwired: 7 in, 2 out]
  n240 = case shown="True" w5 {
    tunnel: "Variant" -> [_ w796]
    tunnel: w2 -> [_ w802]
    tunnel: [w794 w801] -> w7
    tunnel: w3 -> [w794 w800]
    tunnel: w8 -> [w795 w799]
    tunnel: [w795 w798] -> w6
    frame False {
    }
    frame True {
      n241 = call <userlib>:"Get Variant Attributes__ogtk.vi"("error in"=w799, "Variant"=w796) -> ("error out"=w797:errorcluster, "value(s)"=w805:variant[], "names"=w804:string[])  [unwired: 2 in, 1 out]
      n242 = Array Size(array=w804) -> (size(s)=w803:i32)
      n243 = case shown="Default" w803 {
        tunnel: w797 -> [w806 w823]
        tunnel: w805 -> [_ w821]
        tunnel: w804 -> [_ w817]
        tunnel: w802 -> [_ w811]
        tunnel: w800 -> [w807 w810]
        tunnel: [w807 w816] -> w801
        tunnel: [w806 w822] -> w798
        frame 0 {
        }
        frame Default {
          # "Has Attributes"
          n244 = Unbundle By Name(w810) -> ("Tree Ref"=w809:refnum<vi>)
          n245 = invoke on="AddItem" class="Tree" method="Edit Tree Items.Add Item"(reference=w809, error in=w823, "Parent Tag"=w811, "Child Position"=-1, "Left Cell"="Attributes" ("Left Cell String")) -> (reference out=w808:refnum<vi>, error out=w820:errorcluster, "Edit Tree Items:Add Item"=w814:string)  [unwired: 4 in, 6 out]
          n246 = for {
            tunnel: w821 -> [w827] mode=indexing
            tunnel: [w830] -> w818 mode=indexing
            tunnel: w817 -> [w826] mode=indexing
            shift-right: [w831] -> w819
            shift-left: w820 -> [w832]
            n247 = call <vilib>:"GetTypeInfo.vi"("Variant"=w827) -> ("Type Enum"=w829:T7)  [unwired: 6 in, 4 out]
            n248 = case shown="\"Invalid Type\", \"Void\"" w829 {
              tunnel: [w834 w836] -> w828
              tunnel: w827 -> [w834 w839]
              tunnel: w826 -> [w833 w835]
              tunnel: [w833 w835] -> w825
              frame Default {
              }
              frame "Invalid Type", "Void" {
                n249 = Get Variant Attribute(Variant=w839) -> (names=w838:string[], values=w837:variant[])  [unwired: 3 in, 2 out]
                n250 = for {
                  tunnel: w838 -> [w843] mode=indexing
                  tunnel: w837 -> [w842] mode=indexing
                  shift-right: [w840] -> w836
                  shift-left: w835 -> [w841]
                  n251 = Set Variant Attribute(Variant=w841, name=w843, value=w842) -> (Variant out=w840:variant)  [unwired: 1 in, 2 out]
                }
              }
            }
            n252 = call <userlib>:"Set Data Name__ogtk.vi"("error in (no error)"=w832, "Data Name"=w825, "Data"=w828) -> ("error out"=w831:errorcluster, "Renamed Data"=w830:variant)  [unwired: 7 in]
          }
          n253 = property class="Tree"(reference=w808, "Active Item Tag"=w814, "ActiveColNum"=0 ("Active Cell:Active Column Number"), "CellFontColor"=u32 11842740) -> ()  [unwired: 1 in, 2 out]
          n254 = call-dynamic "browseVariantArray.vi"("Array of Variants"=w818, "error in"=w819, "ParentTag"=w814, "VariantProbe.lvclass in"=w810) -> ("error out"=w822:errorcluster, "VariantProbe.lvclass out"=w816:refnum<class "Failures_VariantTree__VP.lvclass">)  [unwired: 4 in]
        }
      }
    }
  }
  "VariantProbe.lvclass out" <- w7
  "error out" <- w6
